vi "Two line search.vi"(0 "Color Mode (Color Threshold 1)":u16(ring)=1 items=["RGB", "HSL", "HSV", "HSI"], 1 "Red or Hue Range (Color Threshold 1)":cluster{"Lower value":i32, "Upper value":i32}={"Lower value"=59, "Upper value"=255}, 2 "Green or Sat Range (Color Threshold 1)":cluster{"Lower value":i32, "Upper value":i32}={"Lower value"=103, "Upper value"=255}, 3 "Blue or Luma or Val or Inten Range (Color Threshold 1)":cluster{"Lower value":i32, "Upper value":i32}={"Lower value"=87, "Upper value"=255}, 4 "Camera Image 3":T1(plugin-control)) -> (20 "Lines (Shape Detection 1)":T2(array[cluster]) {"End Point"."Y" format="%.2f"; "End Point"."X" format="%.2f"; "Start Point"."Y" format="%.2f"; "Start Point"."X" format="%.2f"}, 21 "Lines Calibrated (Shape Detection 1)":T2(array[cluster]) {"End Point"."Y" format="%.2f"; "End Point"."X" format="%.2f"; "Start Point"."Y" format="%.2f"; "Start Point"."X" format="%.2f"}, 22 "Number of Matches (Shape Detection 1)":i32, 23 "Image Out":T1(plugin-control), 27 "error out":errorcluster)   [LabVIEW 2012]
uses:
  <vilib>/vision/NI_Vision_Development_Module.lvlib
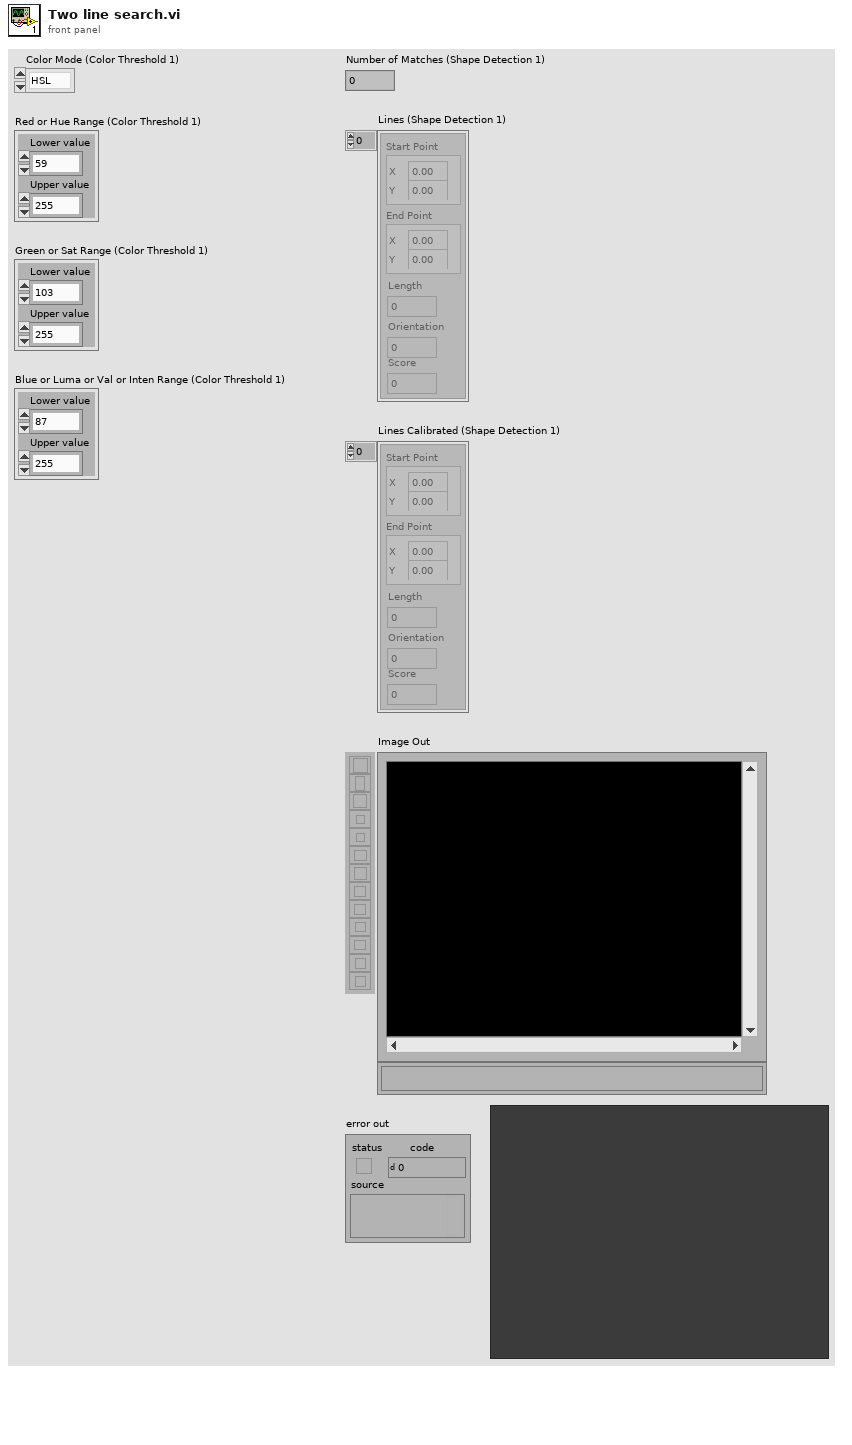
[diagram p1: front panel]
types:
  T1 = typedef "IMAQ Image.ctl" = refnum<image>
  T2 = cluster{"Start Point":cluster{"X":sgl, "Y":sgl}, "End Point":cluster{"X":sgl, "Y":sgl}, "Length":dbl, "Orientation":dbl, "Score":dbl}[]
  T3 = typedef "IMAQ Rectangle" = cluster{"Left":i32, "Top":i32, "Right":i32, "Bottom":i32, "Rotation":dbl}
  T4 = cluster{"Extraction Mode":u32, "Edge Threshold":i32, "Edge Filter Size":u32, "Min Length":i32, "Row Search Step Size":i32, "Col Search Step Size":i32, "Max Endpoint Gap":i32, "Closed":bool, "Subpixel":bool}
  T5 = cluster{"Rotation":bool, "Scale":bool, "Occlusion":bool, "Range Settings":cluster{"Match Constraints":u32, "Min":dbl, "Max":dbl}[]}
  T6 = enum32{"AutoM", "Close", "Dilate", "Erode", "Gradient", "Gradient out", "Gradient in", "Hit miss", "Open", "PClose", "POpen", "Thick", "Thin"}
  T7 = cluster{"histogram":u32[], "Minimal Value":sgl, "Maximal Value":sgl, "Starting Value":sgl, "Interval Width":sgl, "Mean Value":sgl, "Standard  Variation":sgl, "Area (pixels)":i32}
  T8 = typedef "Image Type" = u32
  T9 = cluster{"Global Rectangle":i32[], "Contours":cluster{"ID":enum32{"External", "Internal"}, "Type":u32, "Coordinates":i32[]}[]}
  T10 = typedef "ROI Descriptor" = cluster{"Global Rectangle":i32[], "Contours":cluster{"ID":enum32{"External", "Internal"}, "Type":u32, "Coordinates":i32[]}[]}
  T11 = cluster{"Start Point":cluster{"X":sgl, "Y":sgl}, "End Point":cluster{"X":sgl, "Y":sgl}, "Length":dbl, "Angle":dbl, "Score":dbl}[]
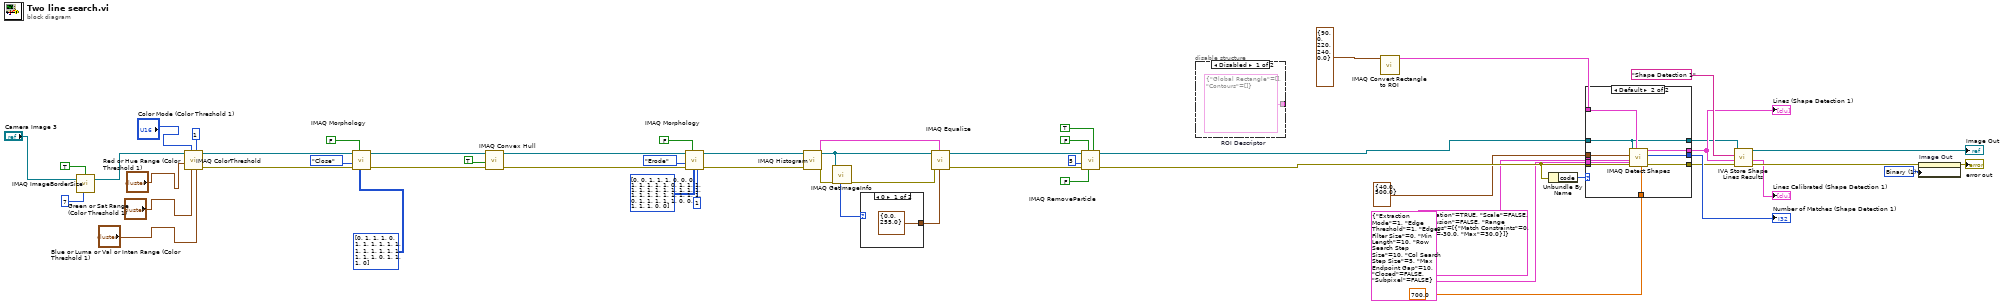
[diagram p0: block diagram]
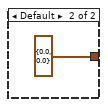
[diagram p4: hidden frame]
diagram:
  w9 = u32 1 items=["Grayscale", "Binary", "Gradient", "Rainbow", "Temperature", "User Defined"] ("Palette")
  n1 = call "IMAQ ImageBorderSize"("Get/Set Status? (Set)"=TRUE, "Image"="Camera Image 3", "Image border size in"=7 ("Border Size")) -> ("Image Out"=w5:T1)  [unwired: 1 in, 2 out]
  n2 = call "IMAQ ColorThreshold"("Blue or Luma or Val or Inten Range"="Blue or Luma or Val or Inten Range (Color Threshold 1)", "Replace Value"=1, "Green or Sat Range"="Green or Sat Range (Color Threshold 1)", "Color Mode"="Color Mode (Color Threshold 1)", "Red or Hue Range"="Red or Hue Range (Color Threshold 1)", "Image Src"=w5) -> ("error out"=w50:errorcluster, "Image Dst Out"=w47:T1)  [unwired: 2 in, 2 out]
  n3 = call "IMAQ Morphology"("Structuring Element"=i32[][] [[0, 1, 1, 1, 0], [1, 1, 1, 1, 1], [1, 1, 1, 1, 1], [1, 1, 1, 1, 1], [0, 1, 1, 1, 0]], "Square/Hexa (Square)"=FALSE, "error in (no error)"=w50, "Operation"=T6."Close", "Image Src"=w47) -> ("error out"=w46:errorcluster, "Image Dst Out"=w45:T1)  [unwired: 2 in, 3 out]
  n4 = call "IMAQ Convex Hull"("error in (no error)"=w46, "Connectivity 4/8 (8)"=TRUE, "Image Src"=w45) -> ("error out"=w43:errorcluster, "Image Dst Out"=w38:T1)  [unwired: 1 in, 6 out]
  n5 = call "IMAQ Morphology"("Number of iterations (1)"=1, "Structuring Element"=i32[][] [[0, 0, 1, 1, 1, 0, 0], [0, 1, 1, 1, 1, 1, 0], [1, 1, 1, 1, 1, 1, 1], [1, 1, 1, 1, 1, 1, 1], [1, 1, 1, 1, 1, 1, 1], [0, 1, 1, 1, 1, 1, 0], [0, 0, 1, 1, 1, 0, 0]], "Square/Hexa (Square)"=FALSE, "error in (no error)"=w43, "Operation"=T6."Erode", "Image Src"=w38) -> ("error out"=w37:errorcluster, "Image Dst Out"=w33:T1)  [unwired: 1 in, 3 out]
  n6 = call "IMAQ Histogram"("error in (no error)"=w37, "Image"=w33) -> ("error out"=w32:errorcluster, "Histogram Report"=w35:T7)  [unwired: 3 in, 5 out]
  n7 = call "IMAQ GetImageInfo"("error in (no error)"=w32, "Image"=w33) -> ("error out"=w31:errorcluster, "Image Type"=w34:T8)  [unwired: 8 out]
  n8 = case shown="0" w34 {
    tunnel: [cluster{"Minimum":sgl, "Maximum":sgl} {"Minimum"=0.0, "Maximum"=255.0} ("Range") cluster{"Minimum":sgl, "Maximum":sgl} {"Minimum"=0.0, "Maximum"=0.0} ("Range")] -> w30
    frame 0 {
    }
    frame Default {
    }
  }
  n9 = call "IMAQ Equalize"("Range"=w30, "Histogram Report"=w35, "error in (no error)"=w31, "Image Src"=w33) -> ("error out"=w36:errorcluster, "Image Dst Out"=w25:T1)  [unwired: 2 in, 4 out]
  n10 = call "IMAQ RemoveParticle"("Connectivity 4/8 (8)"=TRUE, "Low Pass/High Pass (Low)"=FALSE, "Square/Hexa (Square)"=FALSE, "error in (no error)"=w36, "Number of Erosion"=5, "Image Src"=w25) -> ("error out"=w24:errorcluster, "Image Dst Out"=w18:T1)  [unwired: 1 in, 3 out]
  n11 = disable-structure shown="Disabled" {
    disable-tunnel: [w58 _] -> _
    frame Disabled {
      w58 = T9 {"Global Rectangle"=[], "Contours"=[]}  # ROI Descriptor
    }
    frame Enabled {
    }
  }
  n12 = call "IMAQ Convert Rectangle to ROI"("Rectangle"=T3 {"Left"=90, "Top"=0, "Right"=220, "Bottom"=240, "Rotation"=0.0}) -> ("ROI Descriptor"=w1:T10)  [unwired: 8 in, 1 out]
  n13 = Unbundle By Name(w24) -> ("code"=w12:i32)
  n14 = case shown="Default" w12 {
    tunnel: w24 -> [_ w69]
    tunnel: [_ w68] -> w23
    tunnel: T5 {"Rotation"=TRUE, "Scale"=FALSE, "Occlusion"=FALSE, "Range Settings"=[{"Match Constraints"=0, "Min"=-30.0, "Max"=30.0}]} ("Match Options") -> [_ w67]
    tunnel: T4 {"Extraction Mode"=1, "Edge Threshold"=1, "Edge Filter Size"=0, "Min Length"=10, "Row Search Step Size"=10, "Col Search Step Size"=5, "Max Endpoint Gap"=10, "Closed"=FALSE, "Subpixel"=FALSE} ("Curve Parameters") -> [_ w66]
    tunnel: 700.0 ("Minimum match score") -> [_ w65]
    tunnel: cluster{"Min Radius":dbl, "Max Radius":dbl} {"Min Radius"=40.0, "Max Radius"=500.0} ("Line Descriptor") -> [_ w64]
    tunnel: w1 -> [_ w63]
    tunnel: w18 -> [w59 w60]
    tunnel: [_ w62] -> w16
    tunnel: [_ w61] -> w15
    tunnel: [w59 w60] -> w11
    frame -1074396199, -1074396198 {
      # "Discard Coordinate\nSystem Error"
    }
    frame Default {
      n15 = call-poly "IMAQ Detect Shapes"("Minimum match score"=w65, "Curve Parameters"=w66, "ROI Descriptor"=w63, "error in (no error)"=w69, "Match Options"=w67, "Line Descriptor"=w64, "Image"=w60) -> ("error out"=w61:errorcluster, "Number of Matches Returned"=w68:i32, "Lines"=w62:T11)  [unwired: 2 out]
    }
  }
  "Number of Matches (Shape Detection 1)" <- w23
  "Lines (Shape Detection 1)" <- w16
  n16 = call <vilib>:"IVA Store Shape Lines Results.vi"("error in (no error)"=w15, "Lines"=w16, "Step Name"="Shape Detection 1", "Image in"=w11) -> ("error out"=w14:errorcluster, "Lines Calibrated"=→"Lines Calibrated (Shape Detection 1)":T2, "Image dup"=→"Image Out":T1)  [unwired: 5 out]
  n17 = property on="Image Out" class="ImageControl"(error in=w14, "Palette:Palette Type"=w9) -> (error out=→"error out":errorcluster)  [unwired: 1 in, 1 out]
